vi "checkin.vi"(0 "HGF_Reference":refnum<class "HGF_Reference.lvclass">, 2 "Object":refnum<class>, 3 "timeout /ms (-1)":i32=-1, 5 "error in (no error)":errorcluster) -> (14 "dup HGF_Reference":refnum<class "HGF_Reference.lvclass">, 17 "timed out?":bool, 19 "error out":errorcluster)   [LabVIEW 2014, in "HGF_BaseClasses.lvlib" / "HGF_Reference.lvclass"]
doc: "Check in the referenced object.\n\n<B>Attention:</B> You need to check out first!"
uses:
  HGF_Reference.lvclass
  HGF_Reference.lvclass/HGF_Reference.ctl
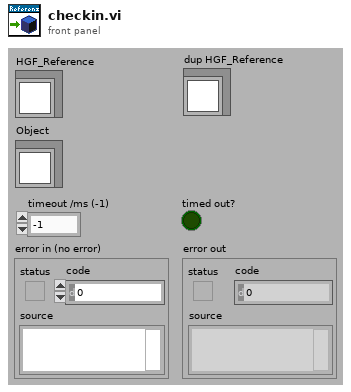
[diagram p1: front panel]
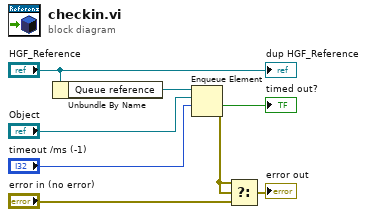
[diagram p0: block diagram]
diagram:
  n1 = Unbundle By Name("HGF_Reference") -> ("Queue reference"=w7:refnum<queue>)
  n2 = Enqueue Element(queue=w7, element="Object", timeout in ms (-1)="timeout /ms (-1)") -> (timed out?=→"timed out?":bool, error out=w8:errorcluster)  [unwired: 1 in, 1 out]
  n3 = Select(t=w8, s=w8, f="error in (no error)") -> (s? t:f=→"error out":errorcluster)
  "dup HGF_Reference" <- "HGF_Reference"
